vi "UsePeanutsProcessing.vi"(11 "Boolean in":refnum<vi>) -> (1 "Process Value":dbl, 2 "Below Threshold":bool, 3 "Above Threshold":bool)   [LabVIEW 2020]
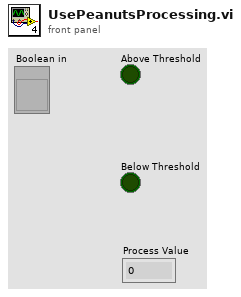
[diagram p1: front panel]
types:
  T1 = enum8{"Enabled", "Disabled", "Disabled and Grayed Out"}
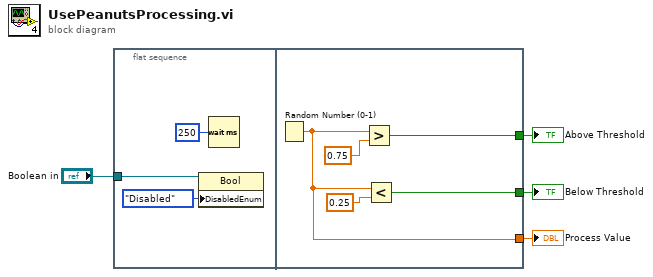
[diagram p0: block diagram]
diagram:
  n1 = flat-sequence {
    tunnel: "Boolean in" -> [w5]
    tunnel: [w12] -> w4
    tunnel: [w9] -> w3
    tunnel: [w8] -> w2
    frame #0 {
      n2 = property on="Property Node" class="Bool"(reference=w5, "DisabledEnum"=T1."Disabled" ("Disabled")) -> ()  [unwired: 1 in, 2 out]
      n3 = Wait (ms)(milliseconds to wait=u32 250) -> ()  [unwired: 1 out]
    }
    frame #1 {
      n4 = Random Number (0-1)() -> (number: 0 to 1=w8:dbl)
      n5 = Greater?(x=w8, y=0.75) -> (0:w12:bool)
      n6 = Less?(x=w8, y=0.25) -> (x < y?=w9:bool)
    }
  }
  "Process Value" <- w2
  "Below Threshold" <- w3
  "Above Threshold" <- w4
